vi "Phasor Universal Semicircle Plot.vi"(6 "Tick Length":dbl=0.02, 8 "Error In":errorcluster, 9 "Show Ticks":bool, 10 "# Decades":i32=4, 11 "Harmonic frequency":dbl[unit]=nan) -> (0 "Error Out":errorcluster, 2 "t Array":dbl[unit][](array[numeric]), 3 "Universal Semi-circle":cluster{"X Array":dbl[], "Y Array":dbl[]})   [LabVIEW 2021, in "Phasor.lvlib"]
uses:
  Phasor.lvlib
  a58c29db-30a8-43e7-8040-62d3e7177082.vi
  <vilib>/Utility/error.llb/Error Cluster From Error Code.vi
  <vilib>/ErrorRing/Error Ring.xnode
panel:
  in  "Log Tick Start":i32=-10
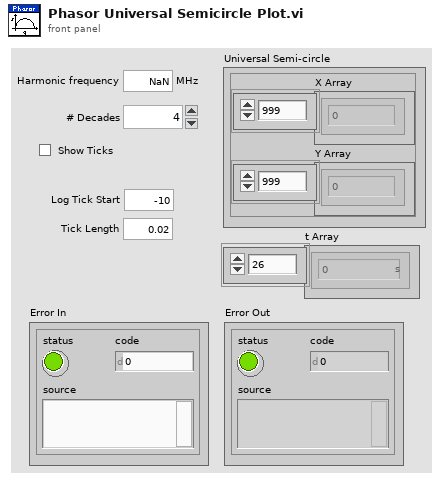
[diagram p1: front panel]
types:
  T1 = typedef "Phasor.lvlib/Phasor (g, s).ctl" = cluster{"g":dbl, "s":dbl}
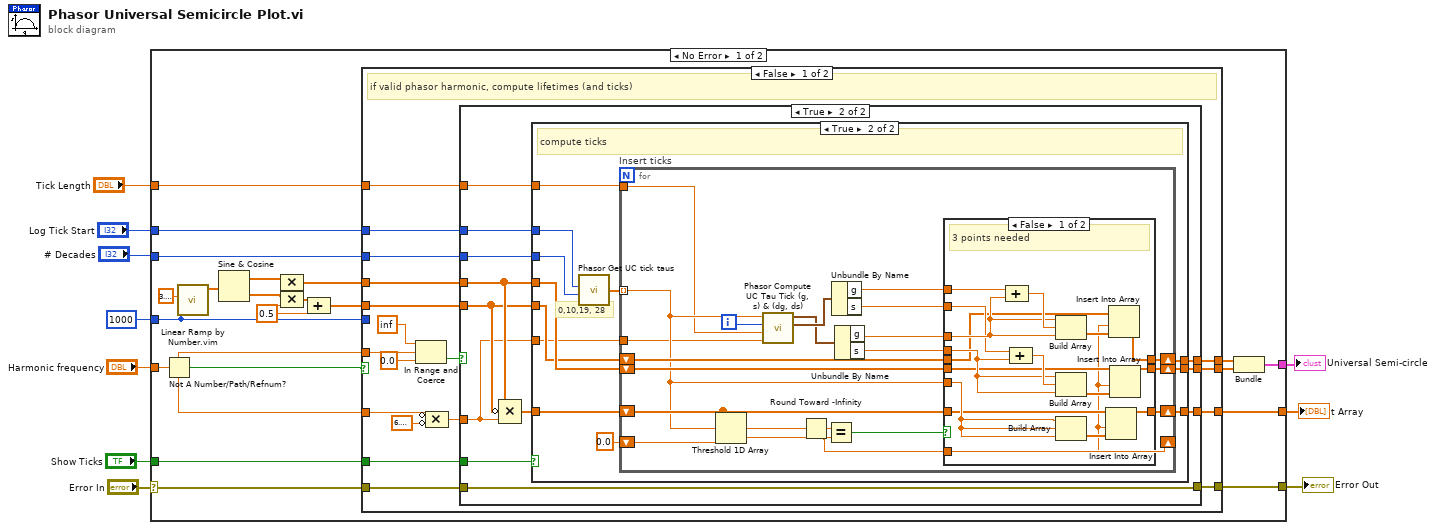
[diagram p0: block diagram]
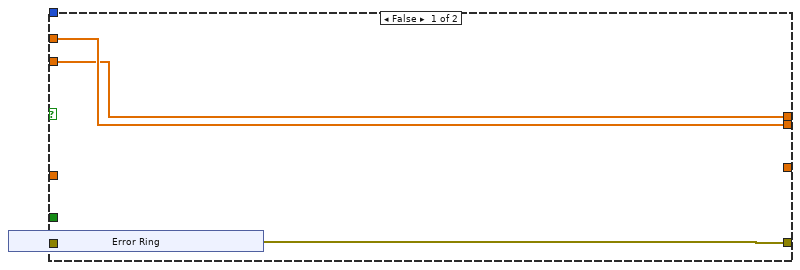
[diagram p2: hidden frame]
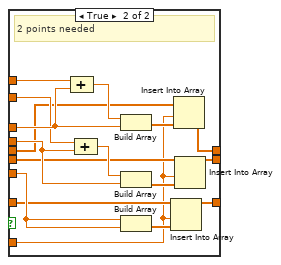
[diagram p4: hidden frame]
diagram:
  n1 = case shown="No Error" "Error In" {
    selector: "Error In" -> [w28 w141]
    tunnel: [w31 _] -> w1
    tunnel: 1000 -> [w25 _]
    tunnel: "Harmonic frequency" -> [w26 _]
    tunnel: "Show Ticks" -> [w29 _]
    tunnel: [w27 w141] -> w6
    tunnel: [w14 _] -> w5
    tunnel: "# Decades" -> [w13 _]
    tunnel: "Log Tick Start" -> [w12 _]
    tunnel: "Tick Length" -> [w11 _]
    frame No Error {
      w20 = 0.5
      n2 = Not A Number/Path/Refnum?(number/path/refnum=w26) -> (NaN/Path/Refnum?=w30:bool)
      n3 = call "Linear Ramp by Number.vim"("# Steps (1)"=w25, "End (1)"=3.141592653589793) -> ("Ramp"=w19:dbl[])  [unwired: 7 in, 2 out]
      n4 = Sine & Cosine(0:w19) -> (1:w21:dbl[], 2:w22:dbl[])
      n5 = Compound Arithmetic op=MULTIPLY(w21, w20) -> (w18:dbl[])
      n6 = Compound Arithmetic op=MULTIPLY(w22, w20) -> (w23:dbl[])
      n7 = Compound Arithmetic op=ADD(w23, w20) -> (w17:dbl[])
      n8 = case shown="False" w30 {
        tunnel: w25 -> [_ _]
        tunnel: w29 -> [w43 _]
        tunnel: w26 -> [w49 _]
        tunnel: w28 -> [w46 w140]
        tunnel: [w44 w140] -> w27
        tunnel: w26 -> [w35 _]
        tunnel: w18 -> [w42 w139]
        tunnel: w17 -> [w41 w138]
        tunnel: [w39 w139] -> w16
        tunnel: [w38 w138] -> w15
        tunnel: [w40 _] -> w14
        tunnel: w13 -> [w37 _]
        tunnel: w12 -> [w36 _]
        tunnel: w11 -> [w32 _]
        frame False {
          # "if valid phasor harmonic, compute lifetimes (and ticks)"
          n9 = In Range and Coerce(upper limit=dbl[unit] inf, x=w49, lower limit=dbl[unit] 0.0) -> (In Range?=w45:bool)  [unwired: 1 out]
          n10 = Compound Arithmetic op=MULTIPLY(invert w35, invert 6.283185307179586) -> (w33:dbl[unit])
          n11 = case shown="True" w45 {
            tunnel: w46 -> [_ w68]
            tunnel: [w52 w68] -> w44
            tunnel: w43 -> [_ w67]
            tunnel: w42 -> [w51 w64]
            tunnel: w41 -> [w50 w63]
            tunnel: w33 -> [_ w57]
            tunnel: [_ w61] -> w40
            tunnel: [w51 w66] -> w39
            tunnel: [w50 w65] -> w38
            tunnel: w37 -> [_ w60]
            tunnel: w36 -> [_ w59]
            tunnel: w32 -> [_ w58]
            frame False {
              n12 = xnode "Error Ring"() -> ("error out"=w52:errorcluster)
            }
            frame True {
              n13 = Compound Arithmetic op=MULTIPLY(w64, invert w63, w57) -> (w62:dbl[unit][])
              n14 = case shown="True" w67 {
                tunnel: w64 -> [w71 w82]
                tunnel: w63 -> [w70 w81]
                tunnel: [w71 w79] -> w66
                tunnel: [w70 w80] -> w65
                tunnel: w62 -> [w69 w83]
                tunnel: [w69 w78] -> w61
                tunnel: w60 -> [_ w73]
                tunnel: w59 -> [_ w74]
                tunnel: w57 -> [_ w76]
                tunnel: w58 -> [_ w75]
                frame False {
                  # "no ticks"
                }
                frame True {
                  # "0,10,19, 28"
                  # "compute ticks"
                  n15 = call "Phasor Get UC tick taus.vi"("Log Tick Start (-10: 100 ps)"=w74, "# Decades (4: 10 ps - 900 ns)"=w73) -> ("Array of taus"=w72:dbl[unit][])  [unwired: 6 in]
                  n16 = for "Insert ticks" {
                    tunnel: w72 -> [w92] mode=indexing
                    shift-right: [w97] -> w78
                    shift-left: w83 -> [w98]
                    shift-right: [w96] -> w79
                    shift-left: w82 -> [w99]
                    shift-right: [w95] -> w80
                    shift-left: w81 -> [w100]
                    shift-right: [w94] -> _
                    shift-left: 0.0 ("start index (0)") -> [w103]
                    tunnel: w76 -> [w90]
                    tunnel: w75 -> [w91]
                    i -> [w93]
                    n17 = Threshold 1D Array(1:w103, 2:w92, 3:w98) -> (0:w94:dbl)
                    n18 = call "Phasor Compute UC Tau Tick (g, s) & (dg, ds).vi"("1/2 pi f"=w90, "Tick Length (0.01)"=w91, "Tick Index"=w93, "tau_i"=w92) -> ("Tick (dg, ds)"=w87:T1, "Tick start (g, s)"=w86:T1)  [unwired: 3 in, 3 out]
                    n19 = Round Toward -Infinity(1:w94) -> (0:w102:dbl)
                    n20 = Equal?(x=w102, y=w94) -> (x = y?=w101:bool)
                    n21 = Unbundle By Name(w87) -> ("g"=w85:dbl, "s"=w84:dbl)
                    n22 = Unbundle By Name(w86) -> ("g"=w89:dbl, "s"=w88:dbl)
                    n23 = case shown="False" w101 {
                      tunnel: w100 -> [w106 w123]
                      tunnel: w99 -> [w110 w127]
                      tunnel: w98 -> [w113 w130]
                      tunnel: w92 -> [w120 w137]
                      tunnel: [w111 w128] -> w97
                      tunnel: [w108 w125] -> w96
                      tunnel: [w104 w121] -> w95
                      tunnel: w89 -> [w118 w135]
                      tunnel: w88 -> [w114 w131]
                      tunnel: w85 -> [w117 w134]
                      tunnel: w84 -> [w115 w132]
                      tunnel: w94 -> [w105 w122]
                      frame False {
                        # "3 points needed"
                        n24 = Compound Arithmetic op=ADD(w117, w118) -> (w119:dbl)
                        n25 = Compound Arithmetic op=ADD(w115, w114) -> (w116:dbl)
                        n26 = Build Array(w118, w119, w118) -> (w107:dbl[])
                        n27 = Build Array(w114, w116, w114) -> (w109:dbl[])
                        n28 = Build Array(w120, w120, w120) -> (w112:dbl[unit][])
                        n29 = Insert Into Array(array=w113, index=w105, new element=w112) -> (w111:dbl[unit][])
                        n30 = Insert Into Array(array=w106, index=w105, new element=w107) -> (w104:dbl[])
                        n31 = Insert Into Array(array=w110, index=w105, new element=w109) -> (w108:dbl[])
                      }
                      frame True {
                        # "2 points needed"
                        n32 = Compound Arithmetic op=ADD(w134, w135) -> (w136:dbl)
                        n33 = Compound Arithmetic op=ADD(w132, w131) -> (w133:dbl)
                        n34 = Build Array(w136, w135) -> (w124:dbl[])
                        n35 = Build Array(w133, w131) -> (w126:dbl[])
                        n36 = Build Array(w137, w137) -> (w129:dbl[unit][])
                        n37 = Insert Into Array(array=w130, index=w122, new element=w129) -> (w128:dbl[unit][])
                        n38 = Insert Into Array(array=w123, index=w122, new element=w124) -> (w121:dbl[])
                        n39 = Insert Into Array(array=w127, index=w122, new element=w126) -> (w125:dbl[])
                      }
                    }
                  }
                }
              }
            }
          }
        }
        frame True {
          # "Ignore phasor harmonic, does not compute ticks"
        }
      }
      n40 = Bundle(w15, w16) -> (w31:cluster{dbl[], dbl[]})  [unwired: 1 in]
    }
    frame Error {
    }
  }
  "Universal Semi-circle" <- w1
  "Error Out" <- w6
  "t Array" <- w5
